vi "module-09-analog-filter.vi"() -> ()   [LabVIEW 2019]
uses:
  <vilib>/Rock Robotics/WPI/ThirdParty/JAS_Junk/TrajLib/LinearFilter_ResetToValue.vi
  <vilib>/Rock Robotics/WPI/ThirdParty/JAS_Junk/TrajLib/LinearFilter_Calculate.vi
  <vilib>/Rock Robotics/WPI/ThirdParty/JAS_Junk/TrajLib/LinearFilter_MovingAverage.vi
  <vilib>/Rock Robotics/WPI/ThirdParty/JAS_Junk/TrajLib/LinearFilter_LowPassBW1.vi
  <vilib>/Rock Robotics/WPI/ThirdParty/JAS_Junk/TrajLib/LinearFilter_LowPassBW2.vi
  <vilib>/Rock Robotics/WPI/ThirdParty/JAS_Junk/TrajLib/LinearFilter_HighPassBW1.vi
  <vilib>/Rock Robotics/WPI/ThirdParty/JAS_Junk/TrajLib/LinearFilter_HighPassBW2.vi
  <vilib>/Rock Robotics/WPI/ThirdParty/JAS_Junk/TrajLib/Trajectory_Library.lvlib
  samples-common-library/Ctrl_Training_Library_Protected/CtrlTrainingLibary_Protected.lvlib
panel:
  in  "Auto / Manual":bool=TRUE
  in  "Noise":bool=TRUE
  in  "Filter Enable":bool=TRUE
  in  "Use White Noise":bool=TRUE
  in  "Tab Control 2":T1(tab)
  out "Avg3":cluster{dbl, dbl, "Value_Output":dbl}(graph)
  out "Avg3 Out Dial":dbl(knob)=-2.895988890827539e-05 scale=-20.0..20.0
  out "Avg3 Out":dbl format="%11.3f"
  out "Med3":cluster{dbl, dbl, "Value_Output":dbl}(graph)
  out "Med3 Out":dbl format="%11.3f"
  out "Med3 Out Dial":dbl(knob)=-2.895988890827539e-05 scale=-20.0..20.0
  out "Avg7":cluster{dbl, dbl, "Value_Output":dbl}(graph)
  out "Avg7 Out":dbl format="%11.3f"
  out "Avg7 Out Dial":dbl(knob)=-2.895988890827539e-05 scale=-20.0..20.0
  out "Med7":cluster{dbl, dbl, "Value_Output":dbl}(graph)
  out "Med7 Out":dbl format="%11.3f"
  out "Med7 Out Dial":dbl(knob)=-2.895988890827539e-05 scale=-20.0..20.0
  out "Lag":cluster{dbl, dbl, "Output_Value":dbl}(graph)
  out "Lag Out":dbl format="%11.3f"
  out "Lag Out Dial":dbl(knob)=-2.895988890827539e-05 scale=-20.0..20.0
  out "Butter 1":cluster{dbl, dbl, "Output_Value":dbl}(graph)
  out "Butter 1 Out":dbl format="%11.3f"
  out "Butter 1 Dial":dbl(knob)=-2.895988890827539e-05 scale=-20.0..20.0
  out "Butter 2":cluster{dbl, dbl, "Output_Value":dbl}(graph)
  out "Butter 2 Out":dbl format="%11.3f"
  out "Butter 2 Dial":dbl(knob)=-2.895988890827539e-05 scale=-20.0..20.0
  out "Duration":dbl format="%11.3f"
  out "Late":dbl format="%11.3f"
  in  "Manual\nInput":dbl(slide) min=-12.0 max=12.0 scale=-12.0..12.0
  out "Raw Noise":dbl(knob)=-2.895988890827539e-05 scale=-20.0..20.0
  out "Raw Noise":dbl format="%11.3f"
  out "Actual Input":dbl(knob)=-2.895988890827539e-05 scale=-20.0..20.0
  out "Actual Input":dbl format="%11.3f"
  in  "Time Const (Sec)":dbl=0.3 min=0.0 step=0.001 format="%10.4f"
  out "Input":cluster{"Manual\nInput":dbl, dbl, "f":dbl}(graph)
  out "Meas Dial":dbl(knob)=-2.895988890827539e-05 scale=-20.0..20.0
  out "Measured Value":dbl format="%11.3f"
  # "Example of Analog FIltering"
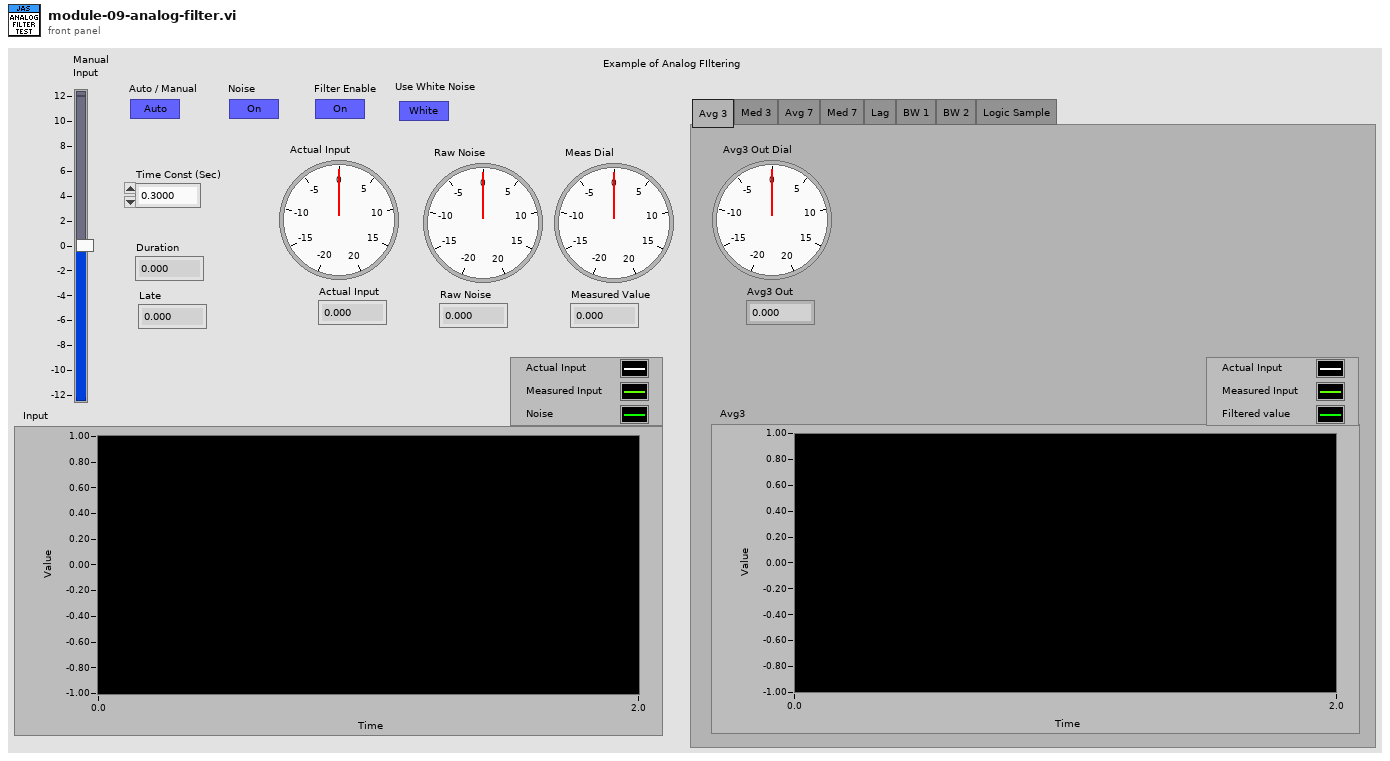
[diagram p1: front panel]
types:
  T1 = enum32{"Avg 3", "Med 3", "Avg 7", "Med 7", "Lag", "BW 1", "BW 2", "Logic Sample"}
  T2 = enum16{"Moving Average", "Low Pass 1st Order Butterworth", "Low Pass 2nd Order Butterworth", "High Pass 1st Order Butterworth", "High Pass 2nd Order Butterworth"}
  T3 = cluster{"Manual\nInput":dbl, dbl, "Output_Value":dbl}
  T4 = cluster{"Manual\nInput":dbl, dbl, "MedianValue":dbl}
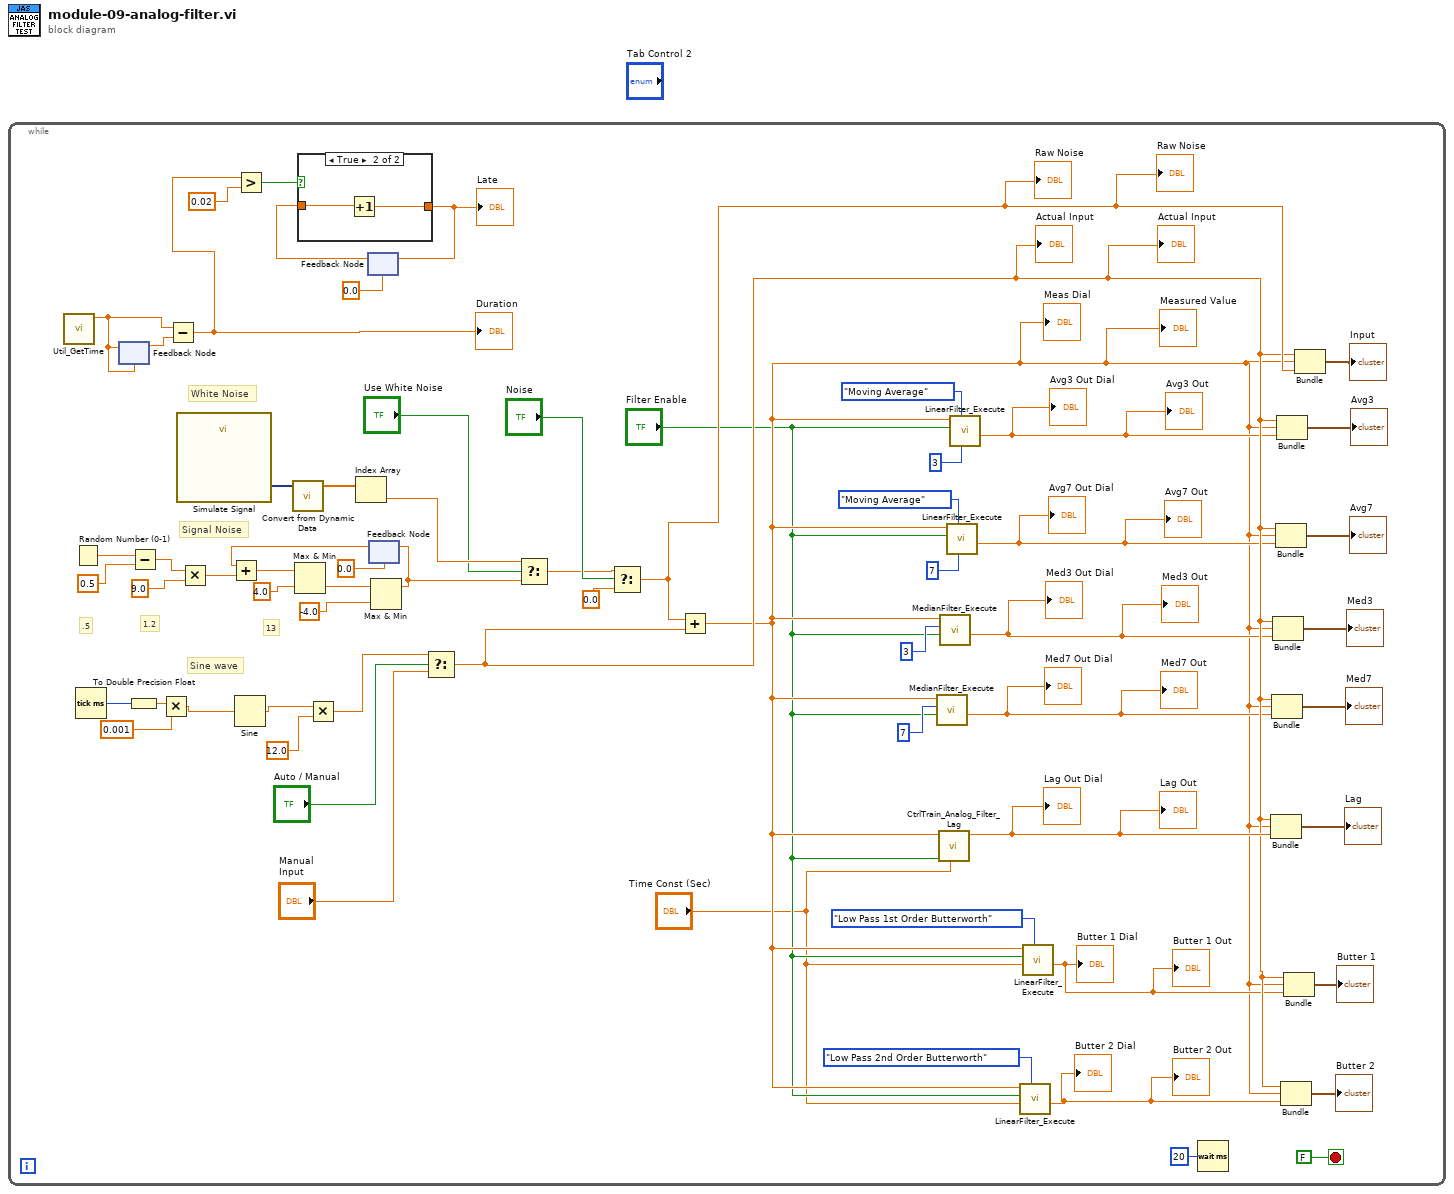
[diagram p0: block diagram]
diagram:
  n1 = while {
    stop <- FALSE stop-if-true
    # "Sine wave"
    # "Signal Noise"
    # "White Noise"
    # "13"
    # "1.2"
    # ".5"
    n2 = call <vilib>:"Util_GetTime.vi"() -> ("FPGA_Time_Seconds"=w5:dbl)  [unwired: 10 in, 1 out]
    n3 = Random Number (0-1)() -> (number: 0 to 1=w61:dbl)
    n4 = Tick Count (ms)() -> (millisecond timer value=w49:u32)
    n5 = feedback-in #1(w5) -> ()
    n6 = feedback #1(w5) -> (w6:dbl)
    n7 = To Double Precision Float(number=w49) -> (double precision float=w50:dbl)
    n8 = Subtract(x=w61, y=0.5) -> (x-y=w57:dbl)
    n9 = Multiply(x=w50, y=0.001) -> (x*y=w47:dbl)
    n10 = Subtract(x=w5, y=w6) -> (x-y=w3:dbl)
    "Duration" <- w3
    n11 = call "Simulate Signal"() -> ("DC with Uniform Noise"=w36:dynamicdata)  [unwired: 14 in, 1 out]
    n12 = Multiply(x=w57, y=9.0) -> (x*y=w56:dbl)
    n13 = Sine(x=w47) -> (sin(x)=w46:dbl)
    n14 = Greater?(x=w3, y=0.02) -> (0:w1:bool)
    n15 = call "Convert from Dynamic Data"("Dynamic Data Type"=w36) -> ("Array"=w35:dbl[])  [unwired: 3 in]
    n16 = Multiply(x=w46, y=12.0) -> (x*y=w42:dbl)
    n17 = Index Array(array=w35) -> (element=w34:dbl)  [unwired: 1 in]
    n18 = feedback #2(0.0) -> (w2:dbl)
    n19 = case shown="True" w1 {
      tunnel: [w67 w69] -> w30
      tunnel: w2 -> [w67 w68]
      frame False {
      }
      frame True {
        n20 = Increment(x=w68) -> (x+1=w69:dbl)
      }
    }
    "Late" <- w30
    n21 = feedback-in #2(w30) -> ()
    n22 = feedback #3(0.0) -> (w58:dbl)
    n23 = Add(x=w58, y=w56) -> (x+y=w60:dbl)
    n24 = Max & Min(x=w60, y=4.0) -> (min(x,y)=w59:dbl)  [unwired: 1 out]
    n25 = Max & Min(x=w59, y=-4.0) -> (max(x,y)=w37:dbl)  [unwired: 1 out]
    n26 = feedback-in #3(w37) -> ()
    n27 = Select(t=w42, s="Auto / Manual", f="Manual\nInput") -> (s? t:f=w26:dbl)
    "Actual Input" <- w26
    "Actual Input" <- w26
    n28 = Select(t=w34, s="Use White Noise", f=w37) -> (s? t:f=w38:dbl)
    n29 = Select(t=w38, s="Noise", f=0.0) -> (s? t:f=w32:dbl)
    "Raw Noise" <- w32
    "Raw Noise" <- w32
    n30 = Add(x=w32, y=w26) -> (x+y=w10:dbl)
    "Measured Value" <- w10
    "Meas Dial" <- w10
    n31 = call <vilib>:"MedianFilter_Execute.vi"("Enable"="Filter Enable", "Samples"=7, "Input Value"=w10) -> ("MedianValue"=w16:dbl)  [unwired: 7 in, 1 out]
    "Med7 Out" <- w16
    "Med7 Out Dial" <- w16
    n32 = call "CtrlTrain_Analog_Filter_Lag.vi"("Time_Const"="Time Const (Sec)", "Enable"="Filter Enable", "Input_Value"=w10) -> ("Output_Value"=w43:dbl)  [unwired: 5 in, 3 out]
    "Lag Out" <- w43
    "Lag Out Dial" <- w43
    n33 = call <vilib>:"MedianFilter_Execute.vi"("Enable"="Filter Enable", "Samples"=3, "Input Value"=w10) -> ("MedianValue"=w19:dbl)  [unwired: 7 in, 1 out]
    "Med3 Out" <- w19
    "Med3 Out Dial" <- w19
    n34 = call <vilib>:"LinearFilter_Execute.vi"("Samples"=7, "Filter Type"=T2."Moving Average", "Enable"="Filter Enable", "Input"=w10) -> ("Output"=w20:dbl)  [unwired: 6 in, 1 out]
    "Avg7 Out" <- w20
    "Avg7 Out Dial" <- w20
    n35 = call <vilib>:"LinearFilter_Execute.vi"("Samples"=3, "Filter Type"=T2."Moving Average", "Enable"="Filter Enable", "Input"=w10) -> ("Output"=w23:dbl)  [unwired: 6 in, 1 out]
    "Avg3 Out" <- w23
    "Avg3 Out Dial" <- w23
    n36 = call <vilib>:"LinearFilter_Execute.vi"("Filter Type"=T2."Low Pass 2nd Order Butterworth", "TimeConstant"="Time Const (Sec)", "Enable"="Filter Enable", "Input"=w10) -> ("Output"=w8:dbl)  [unwired: 6 in, 1 out]
    "Butter 2 Out" <- w8
    "Butter 2 Dial" <- w8
    n37 = call <vilib>:"LinearFilter_Execute.vi"("Filter Type"=T2."Low Pass 1st Order Butterworth", "TimeConstant"="Time Const (Sec)", "Enable"="Filter Enable", "Input"=w10) -> ("Output"=w14:dbl)  [unwired: 6 in, 1 out]
    "Butter 1 Out" <- w14
    "Butter 1 Dial" <- w14
    n38 = Wait (ms)(milliseconds to wait=u32 20) -> ()  [unwired: 1 out]
    n39 = Bundle("Manual\nInput"=w26, w10, "Output_Value"=w43) -> (→"Lag":T3)  [unwired: 1 in]
    n40 = Bundle("Manual\nInput"=w26, w10, "MedianValue"=w16) -> (→"Med7":T4)  [unwired: 1 in]
    n41 = Bundle("Manual\nInput"=w26, w10, "MedianValue"=w19) -> (→"Med3":T4)  [unwired: 1 in]
    n42 = Bundle("Manual\nInput"=w26, w10, "Output"=w20) -> (→"Avg7":cluster{"Manual\nInput":dbl, dbl, "Output":dbl})  [unwired: 1 in]
    n43 = Bundle("Manual\nInput"=w26, w10, "Output"=w23) -> (→"Avg3":cluster{"Manual\nInput":dbl, dbl, "Output":dbl})  [unwired: 1 in]
    n44 = Bundle("Manual\nInput"=w26, w10, "Output"=w8) -> (→"Butter 2":cluster{"Manual\nInput":dbl, dbl, "Output":dbl})  [unwired: 1 in]
    n45 = Bundle("Manual\nInput"=w26, w10, "Output"=w14) -> (→"Butter 1":cluster{"Manual\nInput":dbl, dbl, "Output":dbl})  [unwired: 1 in]
    n46 = Bundle("Manual\nInput"=w26, w10, "f"=w32) -> (→"Input":cluster{"Manual\nInput":dbl, dbl, "f":dbl})  [unwired: 1 in]
  }
